vi "timeslotsFile.vi"(1 "array of clusters":T1(array[cluster]), 2 "error in":errorcluster) -> (0 "error out":errorcluster)   [LabVIEW 2017]
panel:
  out "size(s) 2":i32
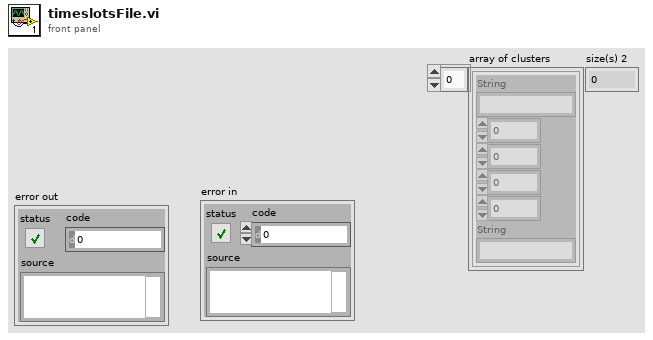
[diagram p1: front panel]
types:
  T1 = cluster{"String":string, i32, i32, u32, u32, "String":string}[]
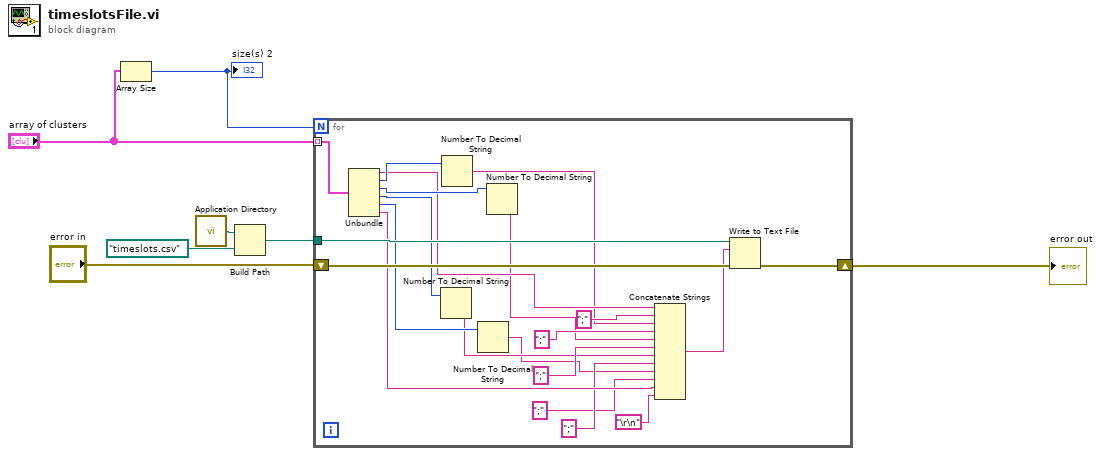
[diagram p0: block diagram]
diagram:
  n1 = Array Size(array="array of clusters") -> (size(s)=w2:i32)
  "size(s) 2" <- w2
  n2 = call <vilib>:"Application Directory.vi"() -> ("Application Directory"=w5:path)
  n3 = Build Path(base path=w5, name or relative path=path "timeslots.csv" ("default name")) -> (appended path=w6:path)
  n4 = for {
    N: w2 -> [_]
    tunnel: w6 -> [w28]
    shift-right: [w26] -> w3
    shift-left: "error in" -> [w27]
    tunnel: "array of clusters" -> [w25] mode=indexing
    n5 = Unbundle(w25) -> ("String"=w20:string, w24:i32, w23:i32, w22:u32, w21:u32, "String"=w13:string)
    n6 = Number To Decimal String(number=w22) -> (decimal integer string=w14:string)  [unwired: 1 in]
    n7 = Number To Decimal String(number=w24) -> (decimal integer string=w18:string)  [unwired: 1 in]
    n8 = Number To Decimal String(number=w21) -> (decimal integer string=w10:string)  [unwired: 1 in]
    n9 = Number To Decimal String(number=w23) -> (decimal integer string=w16:string)  [unwired: 1 in]
    n10 = Concatenate Strings(w20, ";" ("string"), w18, ";" ("string"), w16, ";" ("string"), w14, ";" ("string"), w10, ";" ("string"), w13, "\r\n") -> (w12:string)
    n11 = Write to Text File(file (use dialog)=w28, text=w12, error in=w27) -> (error out=w26:errorcluster)  [unwired: 1 in, 2 out]
  }
  "error out" <- w3
